vi "GetDiagramStructures.vi"(5 "Diagram":refnum<class "Diagram.lvclass">, 6 "error in":errorcluster, 9 "VI Interpreter in":refnum<class "VI Interpreter.lvclass">) -> (0 "error out":errorcluster, 3 "VI Interpreter out":refnum<class "VI Interpreter.lvclass">, 4 "Diagram out":refnum<class "Diagram.lvclass">)   [LabVIEW 2014, in "Raspberry Pi Compatible Compiler for LabVIEW.lvlib" / "VI Interpreter.lvclass"]
uses:
  VI Interpreter.lvclass
  Diagram/Diagram.lvclass
  Diagram/Diagram.lvclass/Diagram.ctl
  Structure/Structure.lvclass
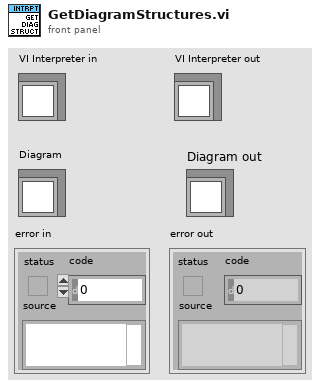
[diagram p1: front panel]
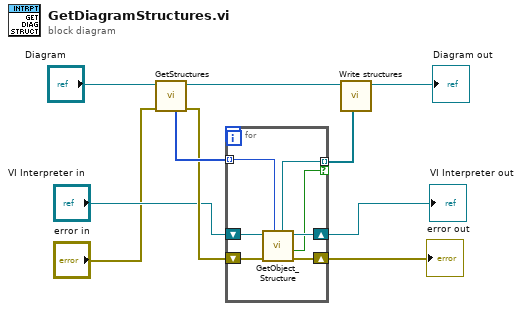
[diagram p0: block diagram]
diagram:
  n1 = call "GetStructures.vi"("error in"="error in", "Diagram in"="Diagram") -> ("error out"=w9:errorcluster, "Diagram out"=w8:refnum<class "Diagram.lvclass">, "structures"=w10:i32[])  [unwired: 5 in]
  n2 = for {
    shift-right: [w14] -> w2
    shift-left: "VI Interpreter in" -> [w17]
    tunnel: w10 -> [w16] mode=indexing
    shift-right: [w15] -> w3
    shift-left: w9 -> [w11]
    tunnel: [w13] -> w7 mode=indexing if=w12
    n3 = call "GetObject_Structure.vi"("UID"=w16, "error in"=w11, "VI Interpreter in"=w17) -> ("error out"=w15:errorcluster, "found"=w12:bool, "VI Interpreter out"=w14:refnum<class "VI Interpreter.lvclass">, "structure"=w13:refnum<class "Structure.lvclass">)  [unwired: 3 in]
  }
  "error out" <- w3
  "VI Interpreter out" <- w2
  n4 = call "Write structures.vi"("structures"=w7, "Diagram in"=w8) -> ("Diagram out"=→"Diagram out":refnum<class "Diagram.lvclass">)  [unwired: 7 in]
